vi "sub vi - Motor Stepper.vi"(0 "?":bool, 8 "Speed Z":dbl=5.0, 11 "Speed XY":dbl=20.0) -> (1 "Z  (7 in - 9 out)":dbl=-378.0, 2 "X  (-600-7000)":dbl=7095.0, 3 "Y (-1000-1000)":dbl=-6372.0)   [LabVIEW 2010]
uses:
  <vilib>/Utility/inputDevices.llb/keyboardAcquire.vi
panel:
  in  "Serial Port":refnum<visa-resource-name>="COM30"
  in  "Motor Current":u16(ring) items=["low", "low-med", "med", "med-high", "high", "very high", "DANGER"]
  # "About this Program:\n     - Controls the Stage Motors using arrows for X and Y axis control and '7' and '9'                \n       for depth control  (Note: '7' goes into the sample and '9' moves out of the sample)"
  # "Motor Parameters"
  # "Motor Position"
  # "F1-Reset Motors and go to Zeros\nF3-Set winding powers\nF2-Step Mode Change"
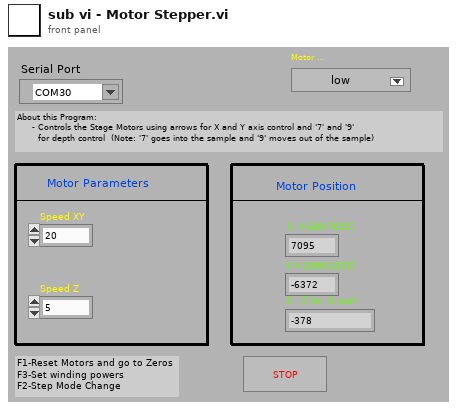
[diagram p1: front panel]
types:
  T1 = enum16{"0", "1", "2", "3", "4", "5", "6", "7", "8", "9", "A", "B", "C", "D", "E", "F", "G", "H", "I", "J", "K", "L", "M", "N", "O", "P", "Q", "R", "S", "T", "U", "V", "W", "X", "Y", "Z", "F1", "F2", "F3", "F4", "F5", "F6", "F7", "F8", "F9", "F10", "F11", "F12", "F13", "F14", "F15", "ADD", "BACK", "BACKSLASH", "CAPITAL", "COMMA", "DECIMAL", "DELETE", "DIVIDE", "DOWN", "END", "EQUALS", "ESCAPE", "GRAVE (`)", "HOME", "INSERT", "LBRACKET", "LCONTROL", "LEFT", "L ALT", "LSHIFT", "LWIN", "MINUS", "MULTIPLY", "NEXT", "NUMLOCK", "NUMPAD_0", "NUMPAD_1", "NUMPAD_2", "NUMPAD_3", "NUMPAD_4", "NUMPAD_5", "NUMPAD_6", "NUMPAD_7", "NUMPAD_8", "NUMPAD_9", "PAUSE", "PERIOD", "PRIOR (PG UP)", "RBRACKET", "RCONTROL", "RETURN", "RIGHT", "R ALT", "RSHIFT", "RWIN", "SCROLL", "SEMICOLON", "SLASH", "SPACE", "SUBTRACT", "TAB", "UP", "ENTER (num pad)", "' (quote)"}[]
  T2 = enum16{"0", "1", "2", "3", "4", "5", "6", "7", "8", "9", "A", "B", "C", "D", "E", "F", "G", "H", "I", "J", "K", "L", "M", "N", "O", "P", "Q", "R", "S", "T", "U", "V", "W", "X", "Y", "Z", "F1", "F2", "F3", "F4", "F5", "F6", "F7", "F8", "F9", "F10", "F11", "F12", "F13", "F14", "F15", "ADD", "BACK", "BACKSLASH", "CAPITAL", "COMMA", "DECIMAL", "DELETE", "DIVIDE", "DOWN", "END", "EQUALS", "ESCAPE", "GRAVE (`)", "HOME", "INSERT", "LBRACKET", "LCONTROL", "LEFT", "L ALT", "LSHIFT", "LWIN", "MINUS", "MULTIPLY", "NEXT", "NUMLOCK", "NUMPAD_0", "NUMPAD_1", "NUMPAD_2", "NUMPAD_3", "NUMPAD_4", "NUMPAD_5", "NUMPAD_6", "NUMPAD_7", "NUMPAD_8", "NUMPAD_9", "PAUSE", "PERIOD", "PRIOR (PG UP)", "RBRACKET", "RCONTROL", "RETURN", "RIGHT", "R ALT", "RSHIFT", "RWIN", "SCROLL", "SEMICOLON", "SLASH", "SPACE", "SUBTRACT", "TAB", "UP", "ENTER (num pad)", "' (quote)"}
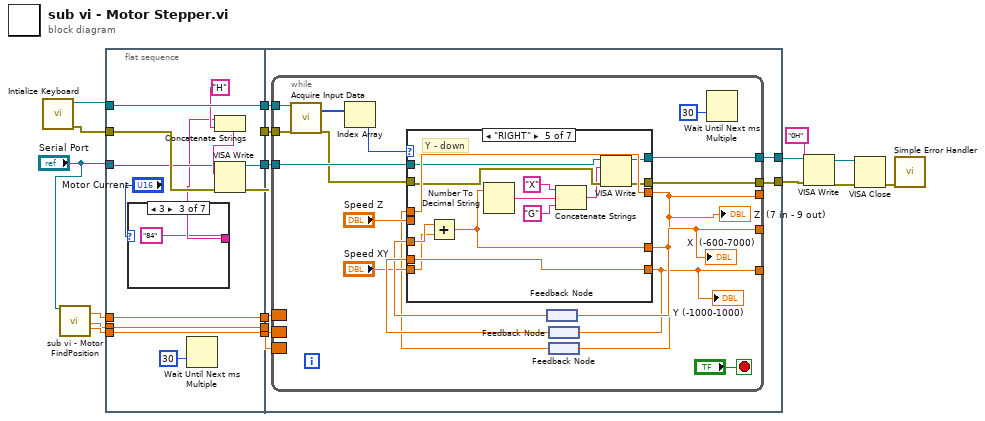
[diagram p0: block diagram]
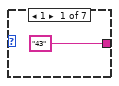
[diagram p2: hidden frame]
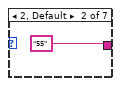
[diagram p3: hidden frame]
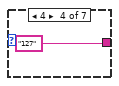
[diagram p4: hidden frame]
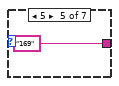
[diagram p5: hidden frame]
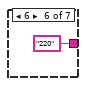
[diagram p6: hidden frame]
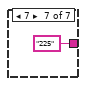
[diagram p7: hidden frame]
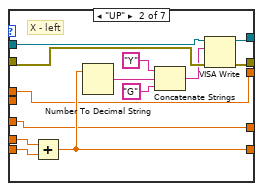
[diagram p9: hidden frame]
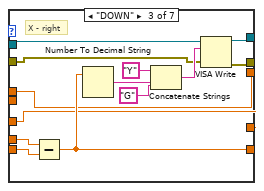
[diagram p10: hidden frame]
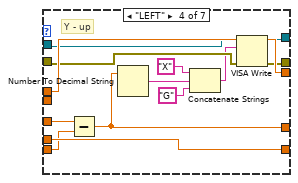
[diagram p11: hidden frame]
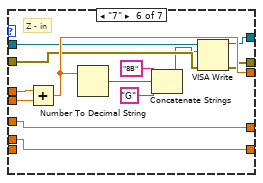
[diagram p12: hidden frame]
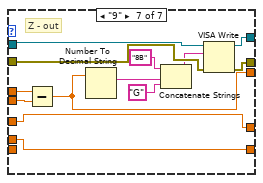
[diagram p13: hidden frame]
diagram:
  n1 = call <vilib>:"Intialize Keyboard.vi"() -> ("error out"=w18:errorcluster, "device ID"=w17:refnum<k1>)  [unwired: 1 in, 9 out]
  n2 = call "sub vi - Motor FindPosition.vi"("VISA resource name"="Serial Port") -> ("X"=w15:dbl, "Y"=w14:dbl, "Z"=w16:dbl)  [unwired: 6 in, 10 out]
  n3 = flat-sequence {
    tunnel: w14 -> [w28]
    tunnel: w15 -> [w29]
    tunnel: w16 -> [w30]
    tunnel: "Serial Port" -> [w23]
    tunnel: w17 -> [w31]
    tunnel: w18 -> [w27]
    tunnel: [w31] -> w13
    tunnel: [w26] -> w12
    tunnel: [w30] -> w11
    tunnel: [w29] -> w10
    tunnel: [w28] -> w9
    tunnel: [w25] -> w8
    tunnel: [w41] -> w5
    tunnel: w13 -> [w46]
    tunnel: w12 -> [w45]
    tunnel: w11 -> [w44]
    tunnel: w10 -> [w43]
    tunnel: w9 -> [w42]
    tunnel: w8 -> [w40]
    tunnel: [w39] -> w2
    frame #0 {
      n4 = case shown="3" "Motor Current" {
        tunnel: ["43" ("string") "55" ("string") "84" ("string") "127" ("string") "169" ("string") "220" ("string") "225" ("string")] -> w19
        frame 1 {
        }
        frame 2, Default {
        }
        frame 3 {
        }
        frame 4 {
        }
        frame 5 {
        }
        frame 6 {
        }
        frame 7 {
        }
      }
      n5 = Wait Until Next ms Multiple(millisecond multiple=u32 30) -> ()  [unwired: 1 out]
      n6 = Concatenate Strings(w19, "H" ("string")) -> (w24:string)
      n7 = VISA Write(VISA resource name=w23, write buffer=w24, error in (no error)=w27) -> (VISA resource name out=w26:refnum<visa-resource-name>, error out=w25:errorcluster)  [unwired: 1 out]
    }
    frame #1 {
      n8 = while {
        tunnel: w40 -> [w64]
        tunnel: w46 -> [w63]
        tunnel: [w54] -> _
        tunnel: [w55] -> _
        border: w42 -> [_]
        border: w43 -> [_]
        border: w44 -> [_]
        tunnel: w45 -> [w53]
        tunnel: [w47] -> _
        tunnel: [w50] -> w41
        tunnel: [w49] -> w39
        stop <- "?" stop-if-true
        n9 = call-poly <vilib>:"Acquire Input Data.vi"("device ID"=w63, "error in (no error)"=w64) -> ("keys pressed"=w60:T1, "error out"=w48:errorcluster)  [unwired: 16 out]
        n10 = Index Array(array=w60) -> (element=w56:T2)  [unwired: 1 in]
        n11 = feedback #1() -> (w58:dbl)
        n12 = feedback #2() -> (w59:dbl)
        n13 = feedback #3() -> (w51:dbl)
        n14 = case shown="\"RIGHT\"" w56 {
          tunnel: w59 -> [w69 w79 w95 w103 w116 w127 w140]
          tunnel: [w69 w77 w94 w103 w116 w127 w140] -> w54
          tunnel: w58 -> [w68 w76 w90 w105 w118 w128 w141]
          tunnel: [w68 w76 w90 w104 w117 w128 w141] -> w55
          tunnel: "Speed XY" -> [_ w78 w89 w101 w114 _ _]
          tunnel: w53 -> [w66 w71 w87 w100 w113 w126 w139]
          tunnel: "Speed Z" -> [_ _ _ _ _ w130 w143]
          tunnel: w51 -> [w67 w75 w88 w102 w115 w129 w144]
          tunnel: [w67 w75 w88 w102 w115 w131 w142] -> w47
          tunnel: [w65 w73 w83 w98 w111 w124 w137] -> w50
          tunnel: [w66 w74 w86 w99 w112 w123 w138] -> w49
          tunnel: w48 -> [w65 w72 w84 w97 w110 w125 w136]
          frame "0", Default {
          }
          frame "UP" {
            # "X - left"
            n15 = Add(x=w79, y=w78) -> (x+y=w77:dbl)
            n16 = Number To Decimal String(number=w77) -> (decimal integer string=w82:string)  [unwired: 1 out]
            n17 = Concatenate Strings("Y", w82, "G") -> (w70:string)
            n18 = VISA Write(VISA resource name=w71, write buffer=w70, error in (no error)=w72) -> (VISA resource name out=w74:refnum<visa-resource-name>, error out=w73:errorcluster)  [unwired: 1 out]
          }
          frame "DOWN" {
            # "X - right"
            n19 = Subtract(x=w95, y=w89) -> (x-y=w94:dbl)
            n20 = Number To Decimal String(number=w94) -> (decimal integer string=w93:string)  [unwired: 1 out]
            n21 = Concatenate Strings("Y", w93, "G") -> (w85:string)
            n22 = VISA Write(VISA resource name=w87, write buffer=w85, error in (no error)=w84) -> (VISA resource name out=w86:refnum<visa-resource-name>, error out=w83:errorcluster)  [unwired: 1 out]
          }
          frame "LEFT" {
            # "Y - up"
            n23 = Subtract(x=w105, y=w101) -> (x-y=w104:dbl)
            n24 = Number To Decimal String(number=w104) -> (decimal integer string=w106:string)  [unwired: 1 out]
            n25 = Concatenate Strings("X", w106, "G") -> (w96:string)
            n26 = VISA Write(VISA resource name=w100, write buffer=w96, error in (no error)=w97) -> (VISA resource name out=w99:refnum<visa-resource-name>, error out=w98:errorcluster)  [unwired: 1 out]
          }
          frame "RIGHT" {
            # "Y - down"
            n27 = Add(x=w118, y=w114) -> (x+y=w117:dbl)
            n28 = Number To Decimal String(number=w117) -> (decimal integer string=w121:string)  [unwired: 1 out]
            n29 = Concatenate Strings("X", w121, "G") -> (w109:string)
            n30 = VISA Write(VISA resource name=w113, write buffer=w109, error in (no error)=w110) -> (VISA resource name out=w112:refnum<visa-resource-name>, error out=w111:errorcluster)  [unwired: 1 out]
          }
          frame "7" {
            # "Z - in"
            n31 = Add(x=w129, y=w130) -> (x+y=w131:dbl)
            n32 = Number To Decimal String(number=w131) -> (decimal integer string=w134:string)  [unwired: 1 out]
            n33 = Concatenate Strings("8B", w134, "G") -> (w122:string)
            n34 = VISA Write(VISA resource name=w126, write buffer=w122, error in (no error)=w125) -> (VISA resource name out=w123:refnum<visa-resource-name>, error out=w124:errorcluster)  [unwired: 1 out]
          }
          frame "9" {
            # "Z - out"
            n35 = Subtract(x=w144, y=w143) -> (x-y=w142:dbl)
            n36 = Number To Decimal String(number=w142) -> (decimal integer string=w147:string)  [unwired: 1 out]
            n37 = Concatenate Strings("8B", w147, "G") -> (w135:string)
            n38 = VISA Write(VISA resource name=w139, write buffer=w135, error in (no error)=w136) -> (VISA resource name out=w138:refnum<visa-resource-name>, error out=w137:errorcluster)  [unwired: 1 out]
          }
        }
        "Y (-1000-1000)" <- w54
        "X  (-600-7000)" <- w55
        "Z  (7 in - 9 out)" <- w47
        n39 = feedback-in #1(w55) -> ()
        n40 = feedback-in #2(w54) -> ()
        n41 = feedback-in #3(w47) -> ()
        n42 = Wait Until Next ms Multiple(millisecond multiple=u32 30) -> ()  [unwired: 1 out]
      }
    }
  }
  n43 = VISA Write(VISA resource name=w2, write buffer="0H", error in (no error)=w5) -> (VISA resource name out=w3:refnum<visa-resource-name>, error out=w4:errorcluster)  [unwired: 1 out]
  n44 = VISA Close(VISA resource name=w3, error in (no error)=w4) -> (error out=w7:errorcluster)
  n45 = call <vilib>:"Simple Error Handler.vi"("error in (no error)"=w7) -> ()  [unwired: 1 in, 8 out]
